vi "P4CMD Check In.vi"(6 "keep checked out? (F)":bool, 7 "advanced options":variant, 8 "error in (no error)":errorcluster, 9 "comment":string, 10 "files":path[](array[path]), 11 "source control reference in":T1) -> (0 "error out":errorcluster, 1 "dialog box cancelled?":bool, 2 "status message":string, 3 "source control reference out":T1)   [LabVIEW 2017, in "NI_SCC_P4CMD.lvlib"]
uses:
  <vilib>/SourceControl/Providers/P4CMD/NI_SCC_P4CMD.lvlib
  <vilib>/SourceControl/sccapi/SCCAPI Refnum.ctl
  <vilib>/SourceControl/Providers/P4CMD/P4CMD Mgr Functions.ctl
  <vilib>/SourceControl/Providers/P4CMD/P4CMD Operations.ctl
  <vilib>/SourceControl/support/SCCSup Message Strings GLBL.vi
  <vilib>/SourceControl/sccapi/NI_SCC.lvlib
panel:
  in  "CList Template":string="Change: %s\n\nClient: %s\n\nUser: %s\n\nStatus: %s\n\nDescription: %s\n\nJobs: %s\n\nFiles: \n%s"
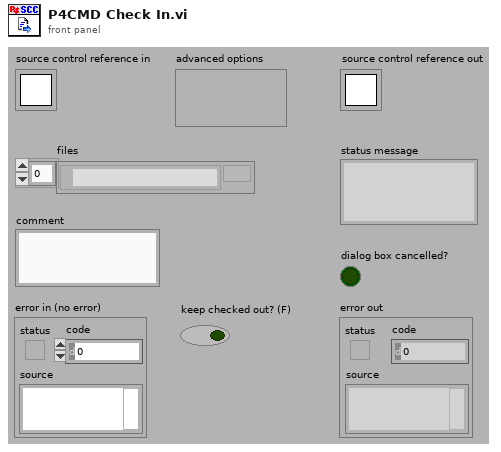
[diagram p1: front panel]
types:
  T1 = typedef "NI_SCC.lvlib/SCCAPI Refnum.ctl" = refnum<k1>
  T2 = typedef "NI_SCC_P4CMD.lvlib/P4CMD Operations.ctl" = enum16{"get all clients", "get all users", "describe changelist", "sync from depot", "open for edit", "submit to depot", "revert", "add to depot", "remove from depot", "print files revisions", "compare client file", "print depot file contents", "list opened files", "get file info", "lock files", "edit changelist spec", "info", "set variables"}
  T3 = typedef "NI_SCC_P4CMD.lvlib/P4CMD Mgr Functions.ctl" = enum16{"Init", "Open", "Set Config Opts", "Initialized?", "IsRefValid?", "Get Config Opts", "Get Global Commands", "Close", "Uninit"}
  T4 = cluster{"changelist":string, "date":string, "client":string, "user":string, "status":string}
  T5 = typedef "NI_SCC_P4CMD.lvlib/P4CMD Advanced Options.ctl" = cluster{"lock files?":bool, "suppress dialogs?":bool}
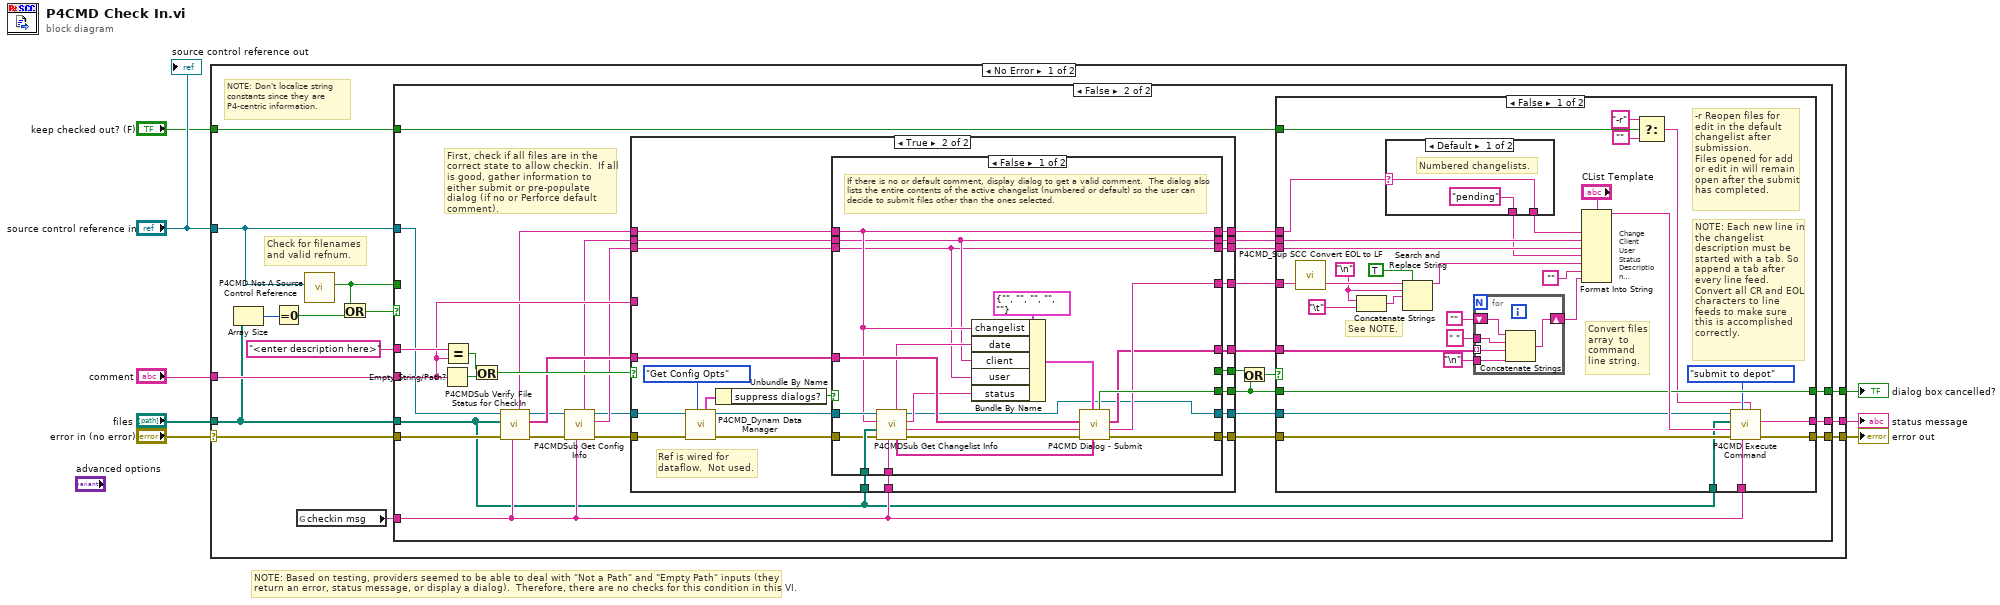
[diagram p0: block diagram]
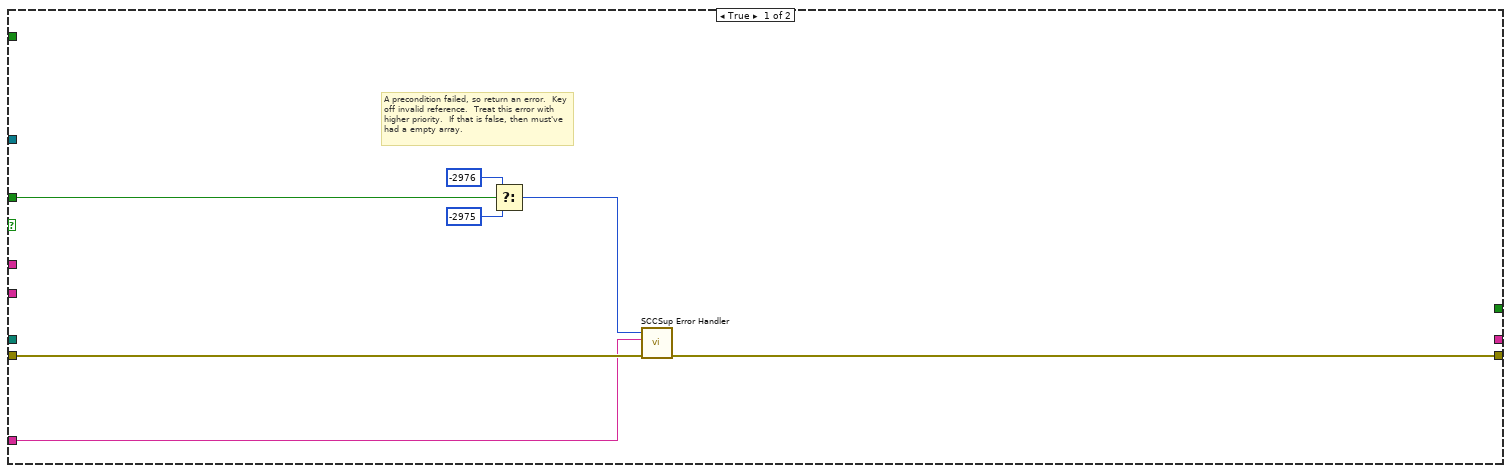
[diagram p2: hidden frame]
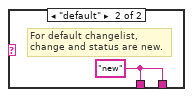
[diagram p3: hidden frame]
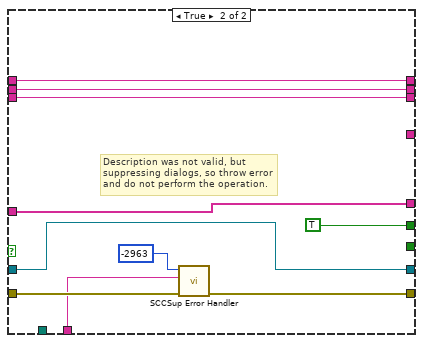
[diagram p6: hidden frame]
diagram:
  # "NOTE: Based on testing, providers seemed to be able to deal with \"Not a Path\" and \"Empty Path\" inputs (they return an error, status message, or display a dialog).  Therefore, there are no checks for this condition in this VI."
  n1 = case shown="No Error" "error in (no error)" {
    selector: "error in (no error)" -> [w13 w162]
    tunnel: [w12 w162] -> w7
    tunnel: "source control reference in" -> [w17 _]
    tunnel: [w20 _] -> w5
    tunnel: "files" -> [w16 _]
    tunnel: "comment" -> [w22 _]
    tunnel: "keep checked out? (F)" -> [w21 _]
    tunnel: [w10 _] -> w1
    frame No Error {
      # "NOTE: Don't localize string constants since they are P4-centric information."
      # "Check for filenames and valid refnum."
      n2 = Array Size(array=w16) -> (size(s)=w19:i32)
      n3 = Equal To 0?(x=w19) -> (x = 0?=w18:bool)
      n4 = global read "SCCSup Message Strings GLBL.vi" "checkin msg"() -> (w11:string)
      n5 = call <vilib>:"P4CMD Not A Source Control Reference.vi"("source control reference in"=w17) -> ("not a source control reference?"=w14:bool)  [unwired: 9 in, 1 out]
      n6 = Or(x=w14, y=w18) -> (x .or. y?=w15:bool)
      n7 = case shown="False" w15 {
        tunnel: w17 -> [_ w46]
        tunnel: [_ w59] -> w20
        tunnel: w16 -> [_ w33]
        tunnel: w22 -> [_ w53]
        tunnel: w21 -> [_ w58]
        tunnel: w14 -> [w27 _]
        tunnel: w13 -> [w26 w45]
        tunnel: [w25 w60] -> w12
        tunnel: w11 -> [w24 w37]
        tunnel: [_ w47] -> w10
        tunnel: "<enter description here>" ("Description:") -> [_ w54]
        frame True {
          # "A precondition failed, so return an error.  Key off invalid reference.  Treat this error with higher priority.  If that is false, then must've had a empty array."
          n8 = Select(t=-2976 ("result"), s=w27, f=-2975 ("result")) -> (s? t:f=w23:i32)
          n9 = call <vilib>:"SCCSup Error Handler.vi"("error in (no error)"=w26, "operation message"=w24, "scc error code"=w23) -> ("error out"=w25:errorcluster)  [unwired: 8 in]
        }
        frame False {
          # "First, check if all files are in the correct state to allow checkin.  If all is good, gather information to either submit or pre-populate dialog (if no or Perforce default comment)."
          n10 = Empty String/Path?(string/path=w53) -> (empty?=w55:bool)
          n11 = Equal?(x=w54, y=w53) -> (x = y?=w52:bool)
          n12 = Or(x=w52, y=w55) -> (x .or. y?=w56:bool)
          n13 = call <vilib>:"P4CMDSub Verify File Status for CheckIn.vi"("operation message"=w37, "error in (no error)"=w45, "files"=w33, "source control reference in"=w46) -> ("error out"=w42:errorcluster, "files (depot format)"=w44:string[], "source control reference out"=w43:T1, "active changelist"=w39:string)  [unwired: 4 in]
          n14 = call <vilib>:"P4CMDSub Get Config Info.vi"("operation message"=w37, "error in (no error)"=w42, "source control reference in"=w43) -> ("error out"=w35:errorcluster, "user"=w40:string, "source control reference out"=w36:T1, "client"=w41:string)  [unwired: 4 in, 1 out]
          n15 = case shown="True" w56 {
            tunnel: w53 -> [w108 _]
            tunnel: w35 -> [w109 w116]
            tunnel: [w109 w131] -> w57
            tunnel: [w108 w127] -> w51
            tunnel: w36 -> [w107 w118]
            tunnel: [w107 w122] -> w50
            tunnel: w41 -> [w106 w129]
            tunnel: w40 -> [w105 w128]
            tunnel: [w106 w113] -> w49
            tunnel: [w105 w114] -> w48
            tunnel: [_ w130] -> w30
            tunnel: w39 -> [w103 w123]
            tunnel: w44 -> [w104 w126]
            tunnel: [w104 w125] -> w38
            tunnel: w37 -> [_ w124]
            tunnel: [w103 w112] -> w34
            tunnel: w33 -> [_ w121]
            tunnel: [_ w110] -> w32
            frame False {
            }
            frame True {
              # "Ref is wired for dataflow.  Not used."
              n16 = call <vilib>:"P4CMD_Dynam Data Manager.vi"("function"=P4CMD_Mgr_Functions."Get Config Opts", "error in (no error)"=w116, "source control reference in"=w118) -> ("error out"=w115:errorcluster, "source control reference out"=w117:T1, "adv cfg options out"=w119:T5)  [unwired: 3 in, 3 out]
              n17 = Unbundle By Name(w119) -> ("suppress dialogs?"=w111:bool)
              n18 = case shown="False" w111 {
                tunnel: [w151 w154] -> w131
                tunnel: [w150 _] -> w130
                tunnel: w129 -> [w133 w160]
                tunnel: w128 -> [w132 w159]
                tunnel: [w147 _] -> w127
                tunnel: w126 -> [w146 w158]
                tunnel: [w145 w158] -> w125
                tunnel: w124 -> [w139 w152]
                tunnel: w123 -> [w134 w161]
                tunnel: [w138 w155] -> w122
                tunnel: w121 -> [w137 _]
                tunnel: w117 -> [w136 w155]
                tunnel: w115 -> [w135 w156]
                tunnel: [w134 w161] -> w112
                tunnel: [w133 w160] -> w113
                tunnel: [w132 w159] -> w114
                tunnel: [_ TRUE] -> w110
                frame False {
                  # "If there is no or default comment, display dialog to get a valid comment.  The dialog also lists the entire contents of the active changelist (numbered or default) so the user can decide to submit files other than the ones selected."
                  n19 = call <vilib>:"P4CMDSub Get Changelist Info.vi"("operation message"=w139, "error in (no error)"=w135, "files"=w137, "changelist"=w134, "source control reference in"=w136) -> ("error out"=w144:errorcluster, "description"=w141:string, "status"=w142:string, "source control reference out"=w138:T1, "changelist files array"=w140:string[], "date"=w143:string)  [unwired: 1 in]
                  n20 = Bundle By Name(cluster=T4 {"changelist"="", "date"="", "client"="", "user"="", "status"=""} ("operation info"), "changelist"=w134, "date"=w143, "client"=w133, "user"=w132, "status"=w142) -> (w148:T4)
                  n21 = call <vilib>:"P4CMD Dialog - Submit.vi"("changelist files"=w140, "operation info"=w148, "error in (no error)"=w144, "description in"=w141, "input files"=w146) -> ("error out"=w151:errorcluster, "description out"=w147:string, "filtered file list"=w145:string[], "dialog box cancelled?"=w150:bool)  [unwired: 3 in]
                }
                frame True {
                  # "Description was not valid, but suppressing dialogs, so throw error and do not perform the operation."
                  n22 = call <vilib>:"SCCSup Error Handler.vi"("error in (no error)"=w156, "operation message"=w152, "scc error code"=-2963 ("error code")) -> ("error out"=w154:errorcluster)  [unwired: 8 in]
                }
              }
            }
          }
          n23 = Or(x=w32, y=w30) -> (x .or. y?=w31:bool)
          n24 = case shown="False" w31 {
            tunnel: [w92 w102] -> w60
            tunnel: [w91 _] -> w59
            tunnel: w58 -> [w71 _]
            tunnel: w37 -> [w90 _]
            tunnel: w57 -> [w89 w102]
            tunnel: w51 -> [w63 _]
            tunnel: w33 -> [w85 _]
            tunnel: w50 -> [w84 _]
            tunnel: w49 -> [w83 _]
            tunnel: w48 -> [w82 _]
            tunnel: [w73 w101] -> w47
            tunnel: w38 -> [w76 _]
            tunnel: w34 -> [w81 _]
            tunnel: w30 -> [w73 w101]
            frame False {
              w66 = "\n" ("Line Feed Constant")
              # "NOTE: Each new line in the changelist description must be started with a tab. So append a tab after every line feed. Convert all CR and EOL characters to line feeds to make sure this is accomplished correctly."
              # "See NOTE."
              # "-r Reopen files for edit in the default changelist after submission.\nFiles opened for add or edit in will remain open after the submit\nhas completed."
              # "Convert files array  to command line string."
              # "Change\nClient\nUser\nStatus\nDescription\nJobs\nFiles"
              n25 = call <vilib>:"P4CMD_Sup SCC Convert EOL to LF.vi"("input string"=w63) -> ("output string"=w67:string)  [unwired: 2 in]
              n26 = Concatenate Strings(w66, "\t") -> (w65:string)
              n27 = case shown="Default" w81 {
                selector: w81 -> [w99 _]
                tunnel: [w99 w100] -> w80
                tunnel: ["pending" ("input 4") w100] -> w79
                frame Default {
                  # "Numbered changelists."
                }
                frame "default" {
                  w100 = "new" ("input 4")
                  # "For default changelist, change and status are new."
                }
              }
              n28 = Search and Replace String(replace all?=TRUE ("replace all? (F)"), input string=w67, search string=w66, replace string=w65) -> (result string=w62:string)  [unwired: 4 in, 3 out]
              n29 = for {
                shift-right: [w97] -> w77
                shift-left: "" -> [w96]
                tunnel: w76 -> [w95] mode=indexing
                tunnel: " " ("string") -> [w94]
                tunnel: "\n" -> [w93]
                n30 = Concatenate Strings(w96, w94, w95, w93) -> (w97:string)
              }
              n31 = Format Into String(format string="CList Template", w80, w83, w82, w79, w62, "", w77) -> (resulting string=w87:string)  [unwired: 2 in, 1 out]
              n32 = Select(t="-r", s=w71, f="") -> (s? t:f=w68:string)
              n33 = call <vilib>:"P4CMD Execute Command.vi"("optional operation parameters"=w68, "operation message"=w90, "p4 operation"=P4CMD_Operations."submit to depot", "error in (no error)"=w89, "input string"=w87, "files"=w85, "source control reference in"=w84) -> ("error out"=w92:errorcluster, "command information"=w91:string)  [unwired: 2 in, 1 out]
            }
            frame True {
              # "Don't perform the operation if user cancelled submit dialog or there was a problem with the description that could not be resolved."
            }
          }
        }
      }
    }
    frame Error {
    }
  }
  "error out" <- w7
  "status message" <- w5
  "dialog box cancelled?" <- w1
  "source control reference out" <- "source control reference in"
